vi "Main Page_InlineAsync.vi"(8 "error in (no error)":errorcluster, 11 "Node Ptr":T1 format="%.0x") -> (0 "error out":errorcluster)   [LabVIEW 2019]
uses:
  <vilib>/NI VeriStand/Custom Device API/Custom Device Item Ref.ctl
  <vilib>/NI VeriStand/Custom Device API/Get Item Property (U16).vi
  <vilib>/NI VeriStand/Custom Device API/Set Item Property (U16).vi
  <vilib>/NI VeriStand/Custom Device API/Custom Device API.lvlib
panel:
  in  "Async Timeout (ms)":u16
  out "Version":string
  in  "SHDocVw.IWebBrowser":refnum<k7>(container)
  in  "Specific Header":cluster{"Section Name":string}={"Section Name"="Custom Device Item Settings"}
  in  "General Header":cluster{"Section Name":string}={"Section Name"="General Custom Device Settings"}
  in  "Description":string
  in  "Name":string
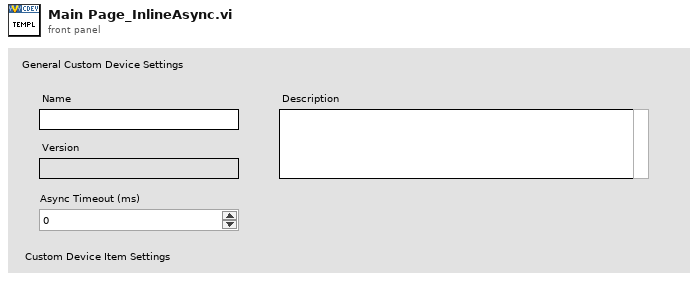
[diagram p1: front panel]
types:
  T1 = typedef "Custom Device API.lvlib/Custom Device Item Ref.ctl" = u64
  T2 = typedef "Custom Device API.lvlib/Custom Device Item Info.ctl" = cluster{"Name":string, "Is Channel":bool, "GUID":string, "Is Waveform":bool}
  T3 = typedef "Custom Device API.lvlib/Custom Device Commands.ctl" = enum16{"Default", "Item renamed", "Shutdown", "Dynamic button pressed"}
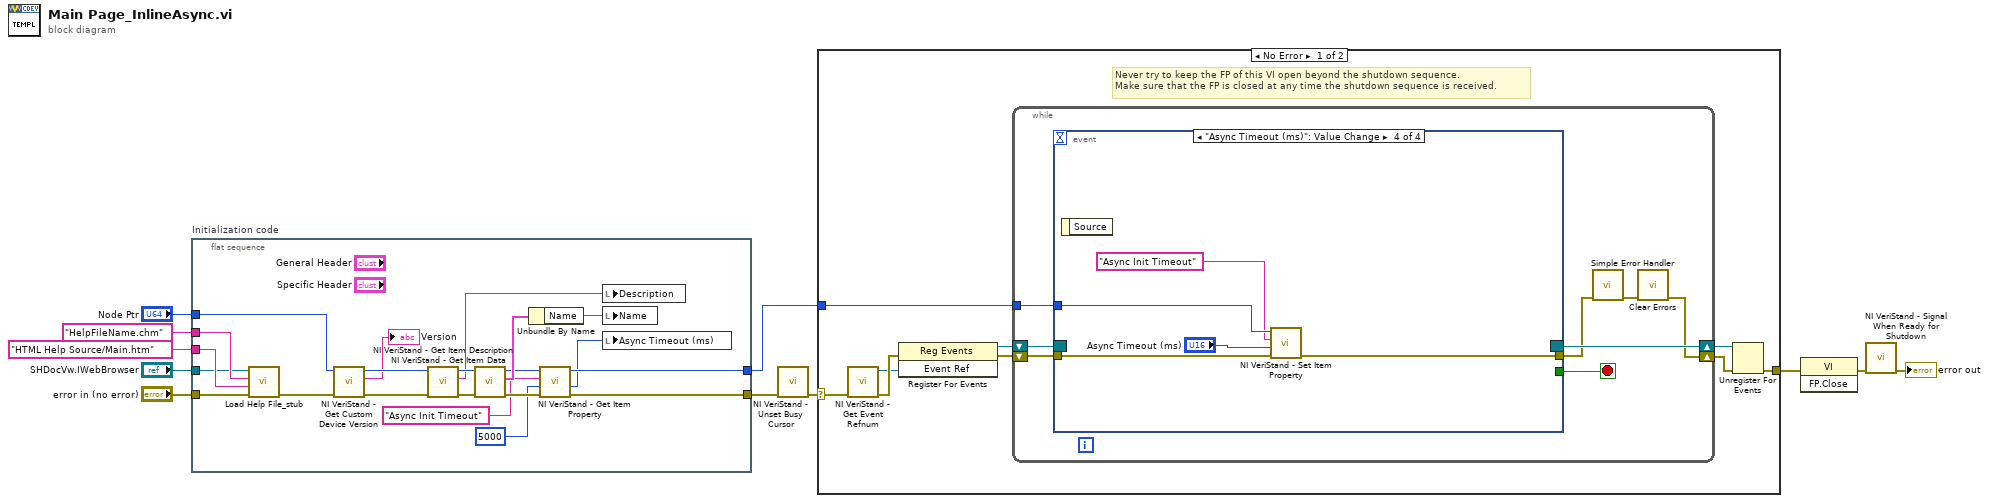
[diagram p0: block diagram]
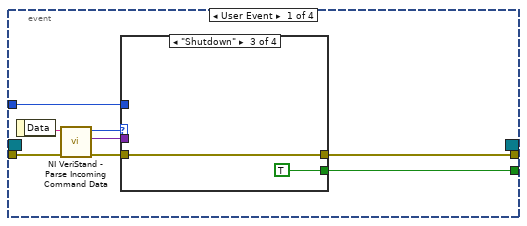
[diagram p2: hidden frame]
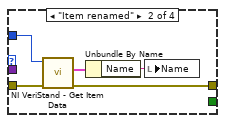
[diagram p4: hidden frame]
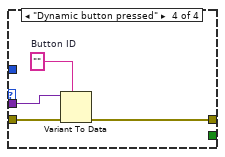
[diagram p5: hidden frame]
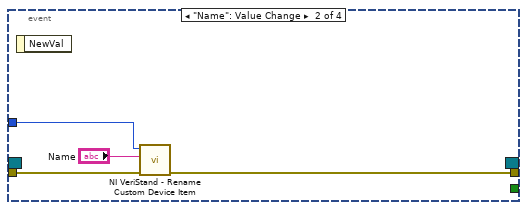
[diagram p6: hidden frame]
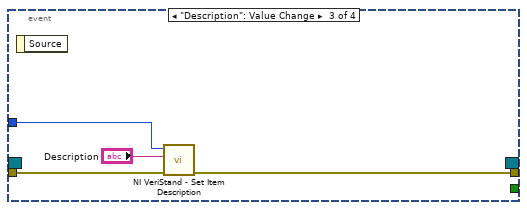
[diagram p7: hidden frame]
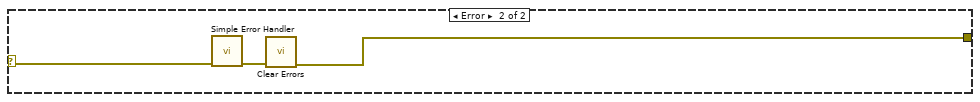
[diagram p8: hidden frame]
diagram:
  n1 = flat-sequence "Initialization code" {
    tunnel: "error in (no error)" -> [w23]
    tunnel: "Node Ptr" -> [w29]
    tunnel: [w17] -> w7
    tunnel: [w15] -> w4
    tunnel: "SHDocVw.IWebBrowser" -> [w19]
    tunnel: "HTML Help Source/Main.htm" ("HTML File") -> [w20]
    tunnel: "HelpFileName.chm" ("CD_CHM_FileName") -> [w21]
    frame #0 {
      n2 = call "Load Help File_stub.vi"("error in (no error)"=w23, "HTML File to Load"=w20, "Main CHM File"=w21, "Browser"=w19) -> ("error out"=w22:errorcluster)  [unwired: 7 in]
      n3 = call <vilib>:"NI VeriStand - Get Custom Device Version.vi"("error in (no error)"=w22, "Device Ref in"=w29) -> ("error out"=w28:errorcluster, "Value"=→"Version":string, "Device Ref out"=w27:T1)  [unwired: 7 in]
      n4 = call <vilib>:"NI VeriStand - Get Item Description.vi"("error in (no error)"=w28, "Item Ref in"=w27) -> ("error out"=w31:errorcluster, "Description"=w24:string, "Item Ref out"=w32:T1)  [unwired: 7 out]
      n5 = call <vilib>:"NI VeriStand - Get Item Data.vi"("error in (no error)"=w31, "Item Ref in"=w32) -> ("error out"=w18:errorcluster, "Item Info"=w30:T2, "Item Ref out"=w16:T1)  [unwired: 7 out]
      n6 = Unbundle By Name(w30) -> ("Name"=w25:string)
      n7 = call-poly <vilib>:"NI VeriStand - Get Item Property.vi"("error in (no error)"=w18, "Default Value"=u16 5000, "Property Name"="Async Init Timeout", "Item Ref in"=w16) -> ("error out"=w17:errorcluster, "Value"=w14:u16, "Item Ref out"=w15:T1)  [unwired: 4 in, 1 out]
      n8 = local write "Description"(w24) -> ()
      n9 = local write "Name"(w25) -> ()
      n10 = local write "Async Timeout (ms)"(w14) -> ()
    }
  }
  n11 = call <vilib>:"NI VeriStand - Unset Busy Cursor.vi"("error in (no error)"=w7) -> ("error out"=w6:errorcluster)  [unwired: 10 out]
  n12 = case shown="No Error" w6 {
    selector: w6 -> [w33 w85]
    tunnel: [w38 w83] -> w11
    tunnel: w4 -> [w34 _]
    frame No Error {
      # "Never try to keep the FP of this VI open beyond the shutdown sequence.\nMake sure that the FP is closed at any time the shutdown sequence is received."
      n13 = call <vilib>:"NI VeriStand - Get Event Refnum.vi"("error in (no error)"=w33) -> ("error out"=w41:errorcluster, "Event Ref"=w37:refnum<user-event>)  [unwired: 9 out]
      n14 = register-events(error in=w41, w37) -> (reference out=w35:refnum<event-registration>, error out=w36:errorcluster)  [unwired: 1 in]
      n15 = while {
        tunnel: w34 -> [w45]
        shift-right: [w42] -> w39
        shift-left: w36 -> [w48]
        shift-right: [w49] -> w40
        shift-left: w35 -> [w47]
        stop <- w46 stop-if-true
        n16 = event shown="[3] \"Async Timeout (ms)\": Value Change" {
          selector: w47 -> [_ _ _ _]
          dyn-events: [_ _ _ _] -> w49
          timeout: _ -> [_ _ _ _]
          tunnel: w48 -> [w57 w73 w76 w82]
          tunnel: [w53 _ _ _] -> w46
          tunnel: [w52 w72 w75 w79] -> w44
          tunnel: w45 -> [w51 w71 w77 w81]
          event User Event {
            n17 = event-data() -> ("Data"=w56:string)  [unwired: 1 out]
            n18 = call <vilib>:"NI VeriStand - Parse Incoming Command Data.vi"("error in (no error)"=w57, "Incoming data"=w56) -> ("error out"=w55:errorcluster, "Outgoing data"=w50:variant, "Action"=w54:T3)  [unwired: 7 out]
            n19 = case shown="\"Shutdown\"" w54 {
              tunnel: w55 -> [w58 w63 w64 w69]
              tunnel: [_ _ TRUE _] -> w53
              tunnel: [w58 w60 w64 w66] -> w52
              tunnel: w51 -> [_ w62 _ _]
              tunnel: w50 -> [_ _ _ w68]
              frame "Default", Default {
              }
              frame "Item renamed" {
                n20 = call <vilib>:"NI VeriStand - Get Item Data.vi"("error in (no error)"=w63, "Item Ref in"=w62) -> ("error out"=w60:errorcluster, "Item Info"=w61:T2)  [unwired: 8 out]
                n21 = Unbundle By Name(w61) -> ("Name"=w59:string)
                n22 = local write "Name"(w59) -> ()
              }
              frame "Shutdown" {
              }
              frame "Dynamic button pressed" {
                w67 = ""  # Button ID
                n23 = Variant To Data(error in=w69, type=w67, Variant=w68) -> (error out=w66:errorcluster)  [unwired: 1 out]
              }
            }
          }
          event "Name": Value Change {
            n24 = event-data() -> ()  [unwired: 2 out]
            n25 = call <vilib>:"NI VeriStand - Rename Custom Device Item.vi"("error in (no error)"=w73, "New Name"="Name", "Item Ref in"=w71) -> ("error out"=w72:errorcluster)  [unwired: 1 in, 7 out]
          }
          event "Description": Value Change {
            n26 = event-data() -> ()  [unwired: 2 out]
            n27 = call <vilib>:"NI VeriStand - Set Item Description.vi"("error in (no error)"=w76, "Description"="Description", "Item Ref in"=w77) -> ("error out"=w75:errorcluster)  [unwired: 8 out]
          }
          event "Async Timeout (ms)": Value Change {
            n28 = event-data() -> ()  [unwired: 2 out]
            n29 = call-poly <vilib>:"NI VeriStand - Set Item Property.vi"("error in (no error)"=w82, "Value"="Async Timeout (ms)", "Property Name"="Async Init Timeout", "Item Ref in"=w81) -> ("error out"=w79:errorcluster)  [unwired: 5 in, 2 out]
          }
        }
        n30 = call <vilib>:"Simple Error Handler.vi"("error in (no error)"=w44) -> ("error out"=w43:errorcluster)  [unwired: 1 in, 7 out]
        n31 = call <vilib>:"Clear Errors.vi"("error in (no error)"=w43) -> ("error out"=w42:errorcluster)  [unwired: 1 in, 5 out]
      }
      n32 = Unregister For Events(event registration refnum=w40, error in=w39) -> (error out=w38:errorcluster)
    }
    frame Error {
      n33 = call <vilib>:"Simple Error Handler.vi"("error in (no error)"=w85) -> ("error out"=w84:errorcluster)  [unwired: 1 in, 7 out]
      n34 = call <vilib>:"Clear Errors.vi"("error in (no error)"=w84) -> ("error out"=w83:errorcluster)  [unwired: 1 in, 5 out]
    }
  }
  n35 = invoke class="VI" method="FP.Close"(error in=w11) -> (error out=w10:errorcluster)  [unwired: 2 in, 2 out]
  n36 = call <vilib>:"NI VeriStand - Signal When Ready for Shutdown.vi"("error in (no error)"=w10) -> ("error out"=→"error out":errorcluster)  [unwired: 10 out]
